vi "Config.Init.vi"(8 "error in":errorcluster) -> (0 "error out":errorcluster)   [LabVIEW 2013]
uses:
  Tma.lib/string.llb/Join array to string.vi
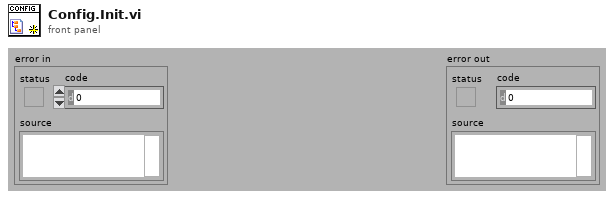
[diagram p1: front panel]
types:
  T1 = enum32{"Bad", "Idle", "Run top level", "Running"}
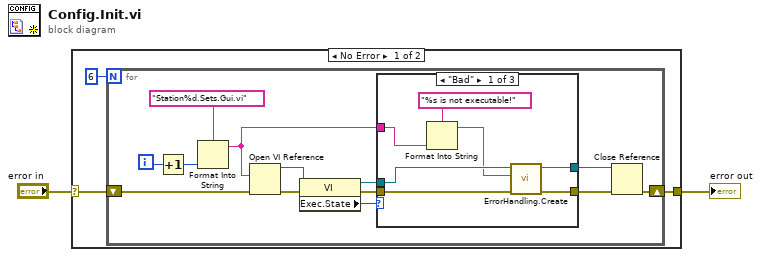
[diagram p0: block diagram]
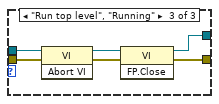
[diagram p3: hidden frame]
diagram:
  n1 = case shown="No Error" "error in" {
    selector: "error in" -> [w5 w33]
    tunnel: [w4 w33] -> w2
    frame No Error {
      n2 = for {
        N: 6 -> [_]
        shift-right: [w10] -> w4
        shift-left: w5 -> [w15]
        i -> [w9]
        n3 = Increment(x=w9) -> (x+1=w6:i32)
        n4 = Format Into String(format string="Station%d.Sets.Gui.vi", w6) -> (resulting string=w7:string)  [unwired: 2 in, 1 out]
        n5 = Open VI Reference(vi path=w7, error in (no error)=w15) -> (vi reference=w17:refnum<vi>, error out=w18:errorcluster)  [unwired: 4 in]
        n6 = property class="VI"(reference=w17, error in=w18) -> (reference out=w14:refnum<vi>, error out=w12:errorcluster, "Exec.State"=w16:T1)
        n7 = case shown="\"Bad\"" w16 {
          tunnel: [w23 w26 w27] -> w11
          tunnel: w12 -> [w24 w26 w32]
          tunnel: [w22 w25 w28] -> w13
          tunnel: w14 -> [w22 w25 w31]
          tunnel: w7 -> [w21 _ _]
          frame "Bad" {
            n8 = Format Into String(format string="%s is not executable!" ("explanation"), w21) -> (resulting string=w19:string)  [unwired: 2 in, 1 out]
            n9 = call "ErrorHandling.Create.vi"("error in"=w24, "explanation"=w19) -> ("error out"=w23:errorcluster)  [unwired: 9 in]
          }
          frame "Idle" {
          }
          frame "Run top level", "Running" {
            n10 = invoke class="VI" method="Abort VI"(reference=w31, error in=w32) -> (reference out=w29:refnum<vi>, error out=w30:errorcluster)  [unwired: 1 in, 1 out]
            n11 = invoke class="VI" method="FP.Close"(reference=w29, error in=w30) -> (reference out=w28:refnum<vi>, error out=w27:errorcluster)  [unwired: 1 in, 1 out]
          }
        }
        n12 = Close Reference(reference=w13, error in (no error)=w11) -> (error out=w10:errorcluster)
      }
    }
    frame Error {
    }
  }
  "error out" <- w2
